vi "bind socket.vi"(8 "error in (no error)":errorcluster, 11 "Socket in":refnum<class "Socket.lvclass">) -> (0 "error out":errorcluster, 3 "Socket out":refnum<class "Socket.lvclass">)   [LabVIEW 2018, in "Socket.lvclass"]
uses:
  Socket.lvclass
  Socket.lvclass/Socket.ctl
  <vilib>/addons/zeromq/zmq_socket.lvclass
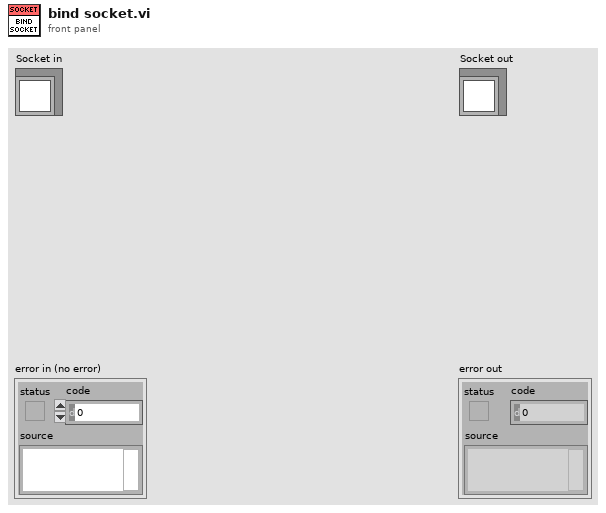
[diagram p1: front panel]
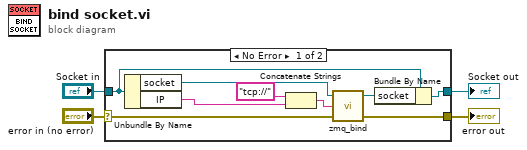
[diagram p0: block diagram]
diagram:
  n1 = case shown="No Error" "error in (no error)" {
    selector: "error in (no error)" -> [w9 w15]
    tunnel: [w8 w15] -> w3
    tunnel: [w11 w14] -> w1
    tunnel: "Socket in" -> [w12 w14]
    frame No Error {
      n2 = Unbundle By Name(w12) -> ("socket"=w13:refnum<class "zmq_socket.lvclass">, "IP"=w6:string)
      n3 = Concatenate Strings("tcp://" ("string"), w6) -> (w7:string)
      n4 = call <vilib>:"zmq_bind.vi"("error in"=w9, "endpoint"=w7, "socket in"=w13) -> ("error out"=w8:errorcluster, "socket out"=w10:refnum<class "zmq_socket.lvclass">)  [unwired: 1 in]
      n5 = Bundle By Name(cluster=w12, "socket"=w10) -> (w11:refnum<class "Socket.lvclass">)
    }
    frame Error {
    }
  }
  "error out" <- w3
  "Socket out" <- w1
